vi "Estrazione fondo - Host.vi"(4 "polynomial order":i32=3, 5 "LowPass Filter: Low cutoff frequency":dbl=20000.0 format="%#_13g", 6 "side points":i32=6, 7 "PolyFitting: Poly Grade":dbl=5.0, 9 "SubtractionType":T1(ring), 10 "error in":errorcluster, 11 "FPGA VI Reference In":refnum<k20>) -> (0 "Fondo Signal":dbl[](graph), 1 "Complete Mean Signal":dbl[](graph), 2 "error out":errorcluster, 3 "FPGA VI Reference Out":refnum<k20>)   [LabVIEW 2014]
uses:
  <vilib>/Analysis/3filter.llb/Filter Passband Type.ctl
  <vilib>/Analysis/3filter.llb/Savitzky-Golay Filter (DBL).vi
  <vilib>/Utility/error.llb/Error Cluster From Error Code.vi
  <vilib>/RVI Host/nirviSupport.llb/nirviErrorClusterFromErrorCode.vi
  <vilib>/rvi/errors/niLvFpgaAdjustHostInterfaceError.vi
  <vilib>/Analysis/3filter.llb/Butterworth Filter (DBL).vi
  <vilib>/rvi/interface/nirviMethod/nirviMethod.xnode
  <vilib>/rvi/errors/niLvFpgaMergeErrorWithErrorCode.vi
  <vilib>/FPGAPlugInAG/Dynamic/niLvFpga_AcknowledgeIrq_Dynamic.vi
  <vilib>/rvi/interface/nirviMethod/StockFPGA_InlinedMethodWaitForSingleIRQ.vi
  <vilib>/FPGAPlugInAG/Dynamic/niLvFpga_WaitOnIrq_Dynamic.vi
  <vilib>/Analysis/NI_AALBase.lvlib
  <vilib>/FPGAPlugInAG/Dynamic/niLvFpga_ReadFifo_Dynamic.vi
  <vilib>/FPGAPlugInAG/Dynamic/niLvFpga_WriteFifo_Dynamic.vi
panel:
  # "SavGolay"
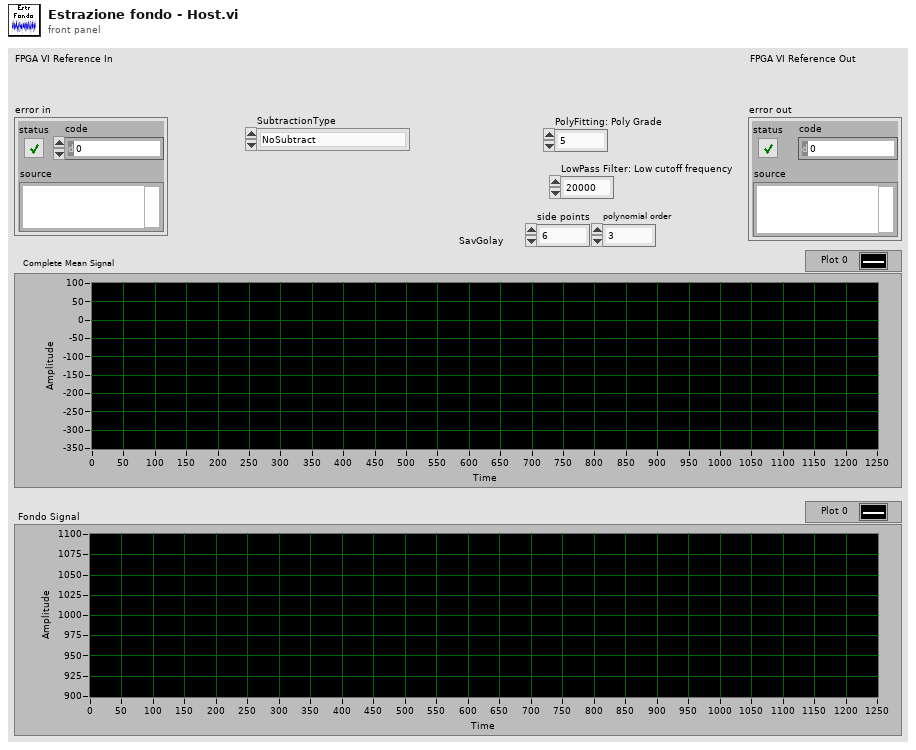
[diagram p1: front panel]
types:
  T1 = enum16{"NoSubtract", "StartingCurve", "LowPass", "PolyFitting", "SavGolay"}
  T2 = typedef "NI_AALBase.lvlib/Filter Passband Type.ctl" = enum32{"Lowpass", "Highpass", "Bandpass", "Bandstop"}
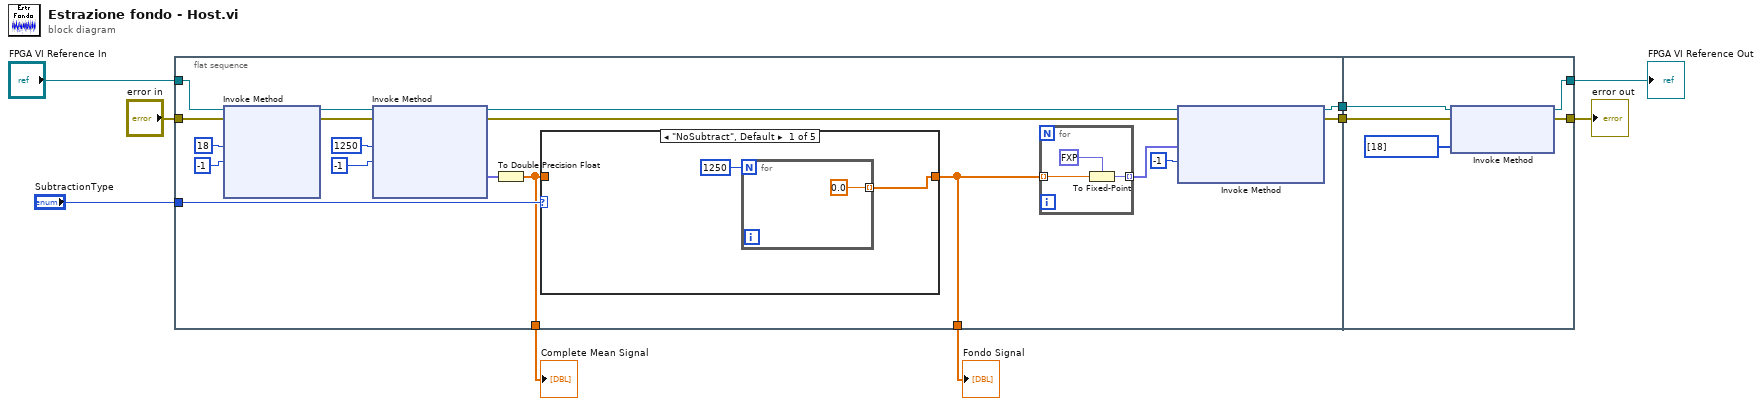
[diagram p0: block diagram]
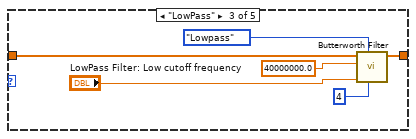
[diagram p3: hidden frame]
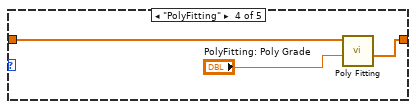
[diagram p4: hidden frame]
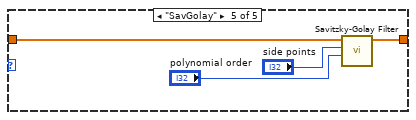
[diagram p5: hidden frame]
diagram:
  n1 = flat-sequence {
    tunnel: [w22] -> w9
    tunnel: [w21] -> w8
    tunnel: "error in" -> [w14]
    tunnel: "FPGA VI Reference In" -> [w13]
    tunnel: "SubtractionType" -> [w12]
    tunnel: [w11] -> w2
    tunnel: [w10] -> w1
    tunnel: w9 -> [w52]
    tunnel: w8 -> [w51]
    tunnel: [w49] -> w4
    tunnel: [w48] -> w5
    frame #0 {
      n2 = xnode "Invoke Method"("FPGA VI Reference In"=w13, "error in"=w14, "IRQ Number(s)"=18, "Timeout (ms)"=-1) -> ("FPGA VI Reference Out"=w17:refnum<k20>, "error out"=w16:errorcluster)  [unwired: 2 out]
      n3 = xnode "Invoke Method"("FPGA VI Reference In"=w17, "error in"=w16, "Number of Elements"=u32 1250, "Timeout (ms)"=-1) -> ("FPGA VI Reference Out"=w25:refnum<k20>, "error out"=w24:errorcluster, "Data"=w18:fxp<+/-,12,12>[])  [unwired: 1 out]
      n4 = To Double Precision Float(number=w18) -> (double precision float=w11:dbl[])
      n5 = case shown="\"NoSubtract\", Default" w12 {
        tunnel: [w28 w31 w33 w38 w43] -> w10
        tunnel: w11 -> [_ w31 w34 w40 w44]
        frame "NoSubtract", Default {
          n6 = for {
            N: 1250 -> [_]
            tunnel: [0.0 ("sampling freq: fs")] -> w28 mode=indexing
          }
        }
        frame "StartingCurve" {
        }
        frame "LowPass" {
          n7 = call-poly <vilib>:"Butterworth Filter.vi"("order"=4, "filter type"=Filter_Passband_Type."Lowpass", "low cutoff freq: fl"="LowPass Filter: Low cutoff frequency", "sampling freq: fs"=40000000.0, "X"=w34) -> ("Filtered X"=w33:dbl[])  [unwired: 3 in, 1 out]
        }
        frame "PolyFitting" {
          n8 = call "Poly Fitting.vi"("Poly Grade"="PolyFitting: Poly Grade", "Signal"=w40) -> ("Poly Signal"=w38:dbl[])  [unwired: 8 in, 1 out]
        }
        frame "SavGolay" {
          n9 = call-poly <vilib>:"Savitzky-Golay Filter.vi"("polynomial order"="polynomial order", "side points"="side points", "X"=w44) -> ("Filtered X"=w43:dbl[])  [unwired: 7 in, 1 out]
        }
      }
      n10 = for {
        tunnel: w10 -> [w47] mode=indexing
        tunnel: [w45] -> w23 mode=indexing
        n11 = To Fixed-Point(fixed-point type=fxp<+/-,12,12> 0.0, number=w47) -> (fixed-point=w45:fxp<+/-,12,12>)
      }
      n12 = xnode "Invoke Method"("FPGA VI Reference In"=w25, "error in"=w24, "Data"=w23, "Timeout (ms)"=-1) -> ("FPGA VI Reference Out"=w22:refnum<k20>, "error out"=w21:errorcluster)  [unwired: 1 out]
    }
    frame #1 {
      n13 = xnode "Invoke Method"("FPGA VI Reference In"=w52, "error in"=w51, "IRQ Number(s)"=i32[] [18]) -> ("FPGA VI Reference Out"=w48:refnum<k20>, "error out"=w49:errorcluster)
    }
  }
  "FPGA VI Reference Out" <- w5
  "error out" <- w4
  "Fondo Signal" <- w1
  "Complete Mean Signal" <- w2
